vi "Drive Straight.vi"   [LabVIEW 2011]
uses:
  jeevan/Global Variables.vi
types:
  T1 = cluster{"Drive Value Output String":string, "Steer Value Output String":string, "Error Out":errorcluster}
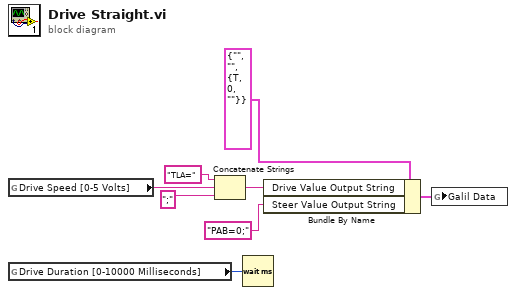
[diagram p0: block diagram]
diagram:
  n1 = global read "Global Variables.vi" "Drive Speed [0-5 Volts]"() -> (w3:string)
  n2 = global read "Global Variables.vi" "Drive Duration [0-10000 Milliseconds]"() -> (w6:u32)
  n3 = Concatenate Strings("TLA=" ("string"), w3, ";" ("string")) -> (w2:string)
  n4 = Wait (ms)(milliseconds to wait=w6) -> ()  [unwired: 1 out]
  n5 = Bundle By Name(cluster=T1 {"Drive Value Output String"="", "Steer Value Output String"="", "Error Out"={"status"=TRUE, "code"=0, "source"=""}} ("Galil Data"), "Drive Value Output String"=w2, "Steer Value Output String"="PAB=0;") -> (w8:T1)
  n6 = global write "Global Variables.vi" "Galil Data"(w8) -> ()
